vi "Set DDG Step Coefficients.vi"(8 "error in (no error)":errorcluster, 9 "p2":dbl, 10 "p1":dbl, 11 "mode":u32) -> (0 "error out":errorcluster, 3 "function return":u32)   [LabVIEW 2014, in "atmcd32d.lvlib"]
doc: "unsigned int WINAPI SetDDGStepCoefficients(at_u32 mode, double p1, double p2);"
uses:
  atmcd32d.lvlib
  atmcd32d.dll
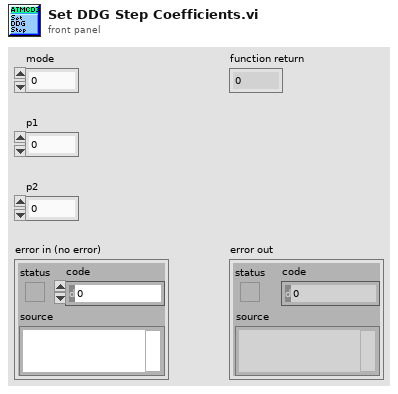
[diagram p1: front panel]
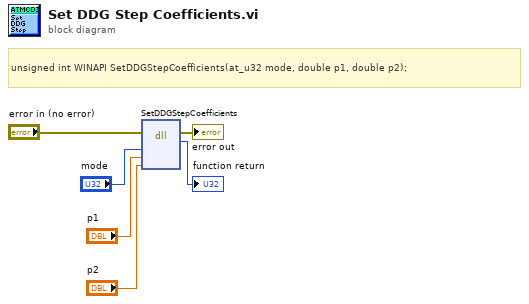
[diagram p0: block diagram]
diagram:
  # "unsigned int WINAPI SetDDGStepCoefficients(at_u32 mode, double p1, double p2);"
  n1 = dll-call lib="C:/Users/Bakir/Documents/Lambda2-Testing/lib/Andorlib/atmcd32d.*" fn="SetDDGStepCoefficients"(error in="error in (no error)", "mode"="mode", "p1"="p1", "p2"="p2") -> (error out=→"error out":errorcluster, →"function return":u32)  [unwired: 5 in, 1 out]
